vi "Calculate Ascan Parameter.vi"(8 "error in (no error)":errorcluster caption="错误输入（无错误）", 10 "data":T1(array[cluster]), 11 "connection reference":T2) -> (0 "error out":errorcluster caption="错误输出")   [LabVIEW 2015, in "Digital Signal Processing.lvlib"]
doc: "该模板用于创建子VI。"
uses:
  Digital Signal Processing.lvlib
  <vilib>/addons/database/Connection.llb/Conn ObjectReference.ctl
  Utility VIs/Utility VIs.lvlib
  <vilib>/Analysis/NI_AALBase.lvlib
  Database Processing/Database Processing.lvlib
  <vilib>/addons/database/NI_Database_API.lvlib
  Digital Image Processing/Digital Image Processing.lvlib
panel:
  # "Busy"
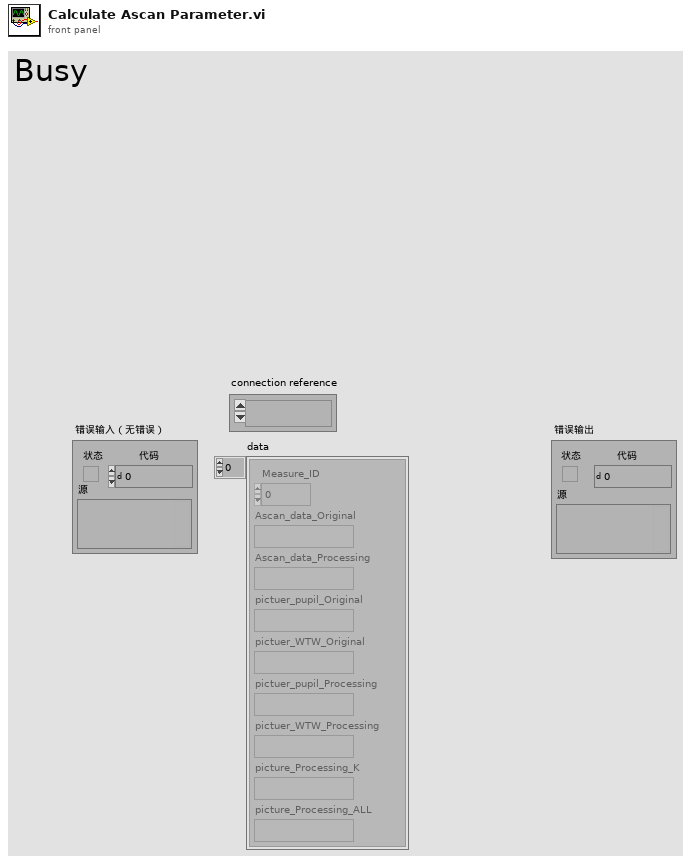
[diagram p1: front panel]
types:
  T1 = cluster{"Measure_ID":i64, "Ascan_data_Original":string, "Ascan_data_Processing":string, "pictuer_pupil_Original":string, "pictuer_WTW_Original":string, "pictuer_pupil_Processing":string, "pictuer_WTW_Processing":string, "picture_Processing_K":string, "picture_Processing_ALL":string}[]
  T2 = typedef "NI_Database_API.lvlib/Conn ObjectReference.ctl" = refnum<k1>
  T3 = cluster{"Measure_ID":i64, "Ascan_data_Original":string, "Ascan_data_Processing":string, "pictuer_pupil_Original":string, "pictuer_WTW_Original":string, "pictuer_pupil_Processing":string, "pictuer_WTW_Processing":string, "picture_Processing_K":string, "picture_Processing_ALL":string}
  T4 = typedef "Digital Signal Processing.lvlib/DSP Configuration.ctl" = cluster{"Sampling Frequency":dbl, "filter type":T5, "RF Filter Low Frequency":dbl, "RF Filter High Frequency":dbl, "RF Filter Taps":i32, "window":T6, "RF window parameter":dbl, "filter type 2":T5, "Demodulated Filter Low Frequency":dbl, "Demodulated Filter HighFrequency":dbl, "Demodulated Filter Order":i32, "SPAN":i32, "Logarithmic Base":dbl, "Noise path":string, "Work position parameter":i32[]}
  T5 = typedef "NI_AALBase.lvlib/Filter Passband Type.ctl" = enum32{"Lowpass", "Highpass", "Bandpass", "Bandstop"}
  T6 = typedef "NI_AALPro.lvlib/windowTd.ctl" = u32
  T7 = cluster{"filter structure":enum32{"IIR 2nd Order", "IIR 4th Order"}, "Reverse Coefficients":dbl[], "Forward Coefficients":dbl[]}
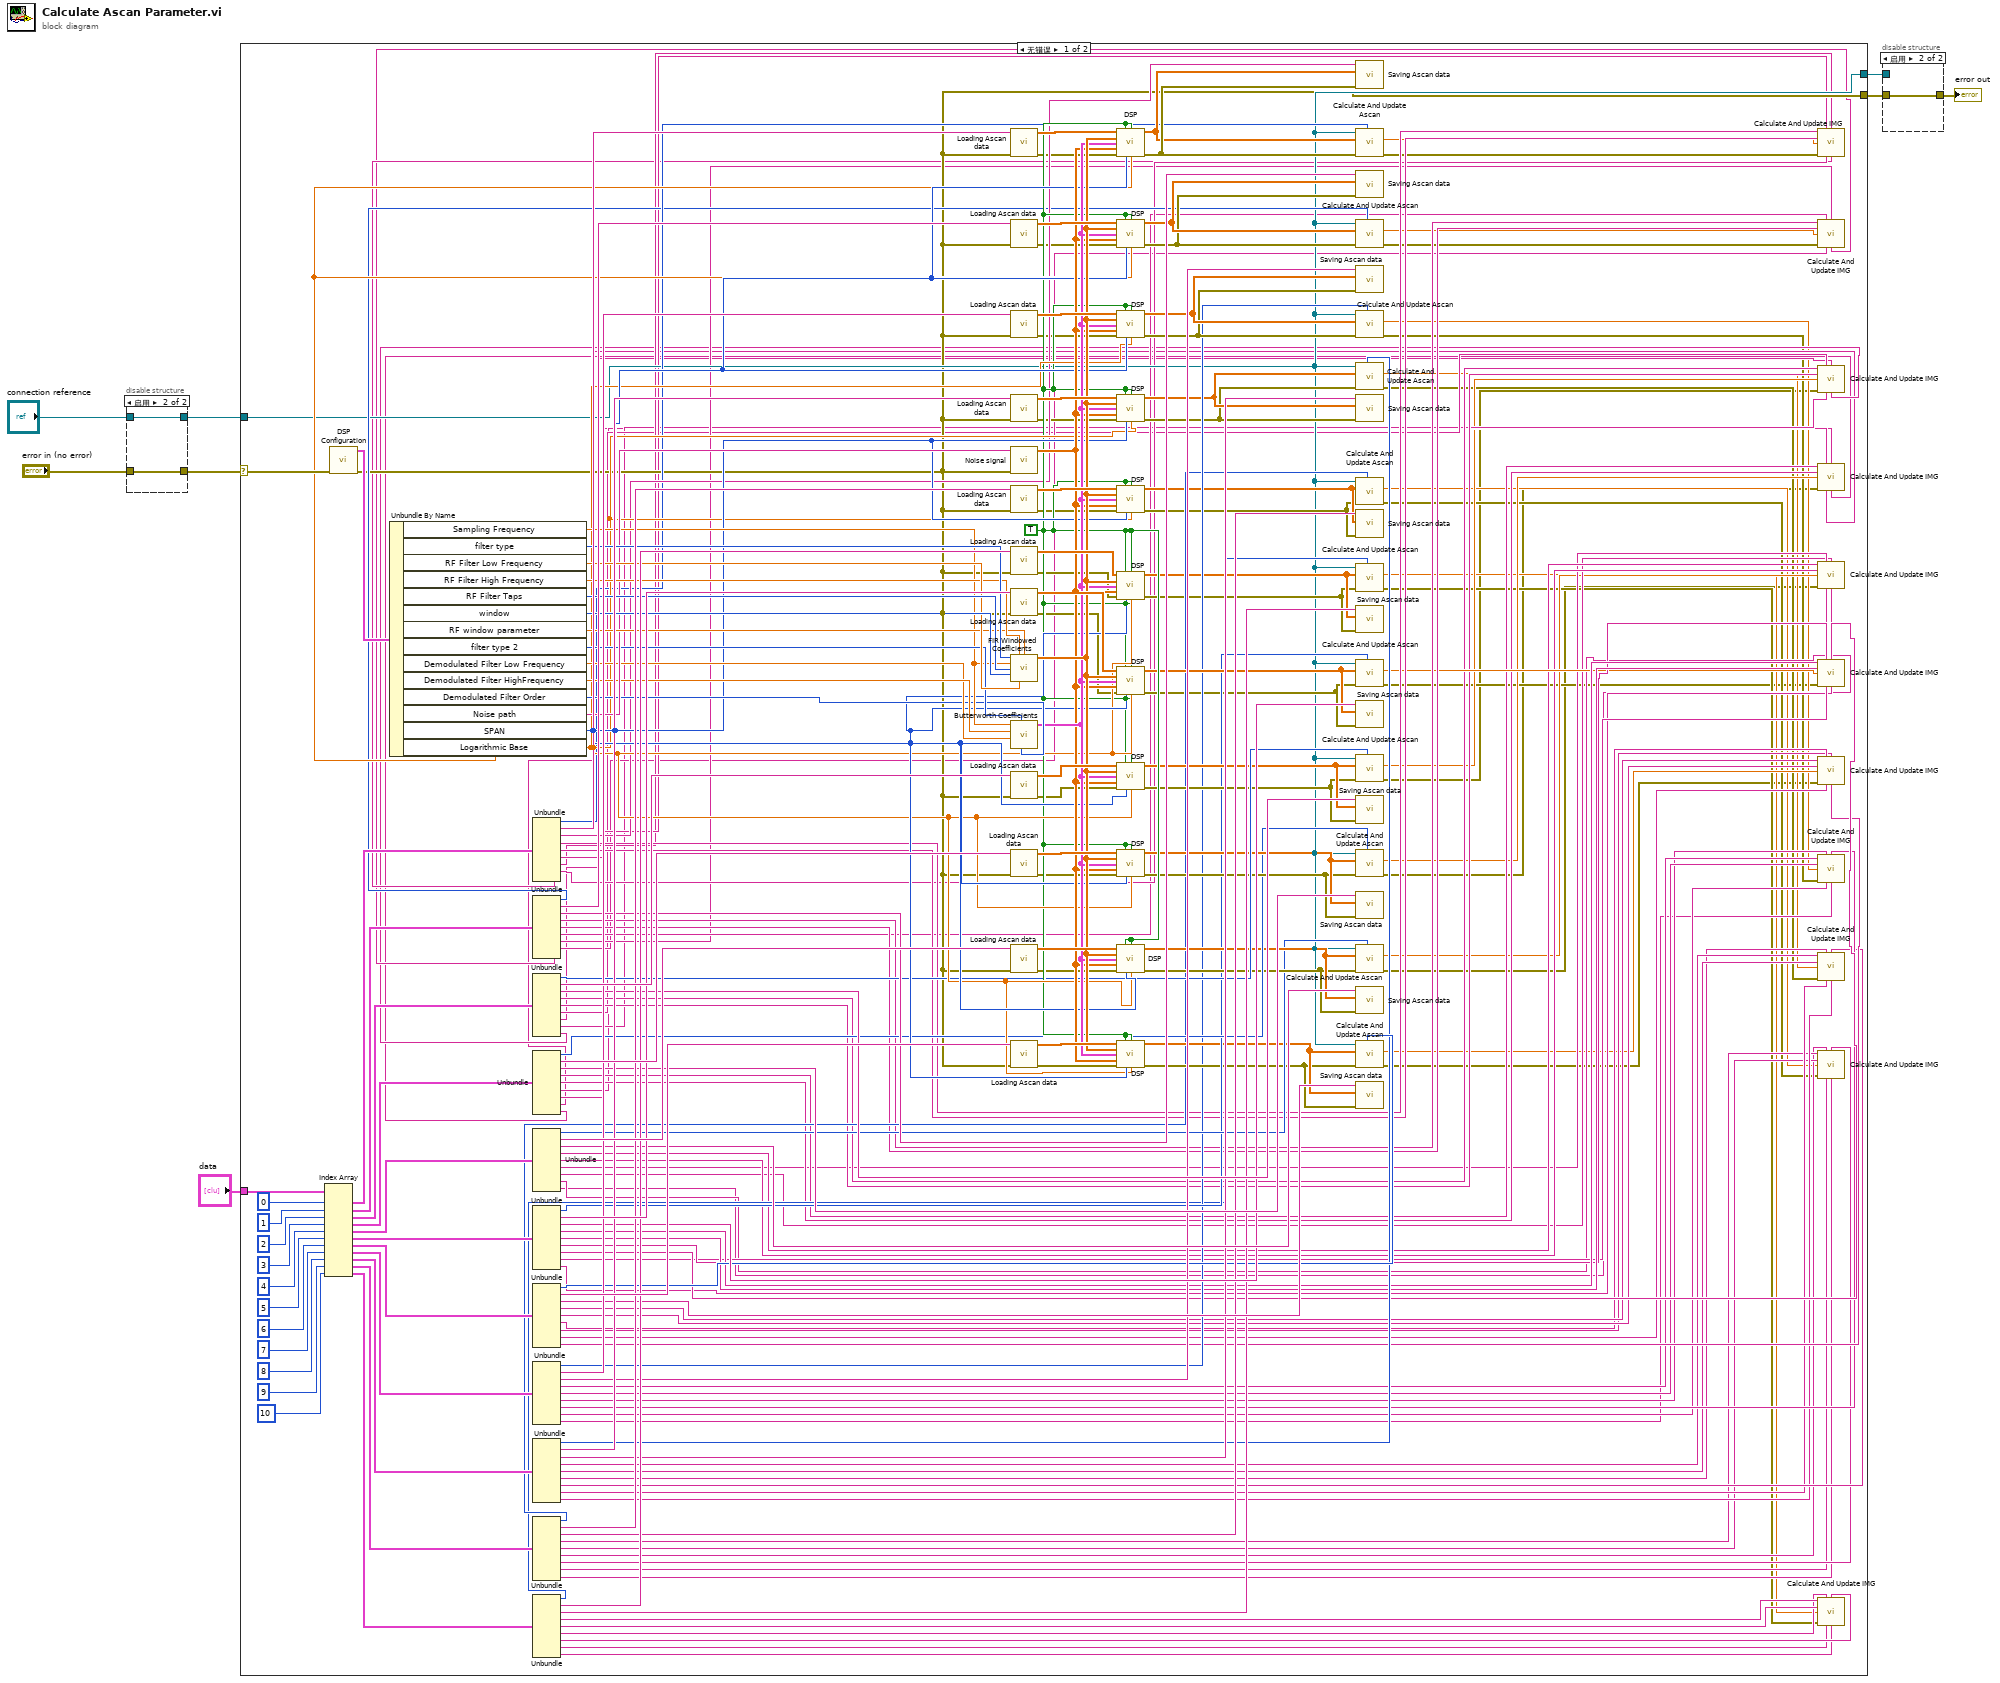
[diagram p0: block diagram]
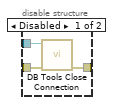
[diagram p2: hidden frame]
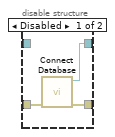
[diagram p3: hidden frame]
diagram:
  n1 = disable-structure shown="启用" {
    disable-tunnel: [w11 w13] -> w8
    disable-tunnel: "error in (no error)" -> [w10 w12]
    disable-tunnel: [w9 w12] -> w6
    disable-tunnel: "connection reference" -> [_ w13]
    frame Disabled {
      n2 = call "Connect Database.vi"("error in (no error)"=w10) -> ("error out"=w9:errorcluster, "connection reference"=w11:T2)  [unwired: 9 in]
    }
    frame Enabled {
    }
  }
  n3 = case shown="无错误" w6 {
    selector: w6 -> [w166 w225]
    tunnel: [w102 w225] -> w4
    tunnel: "data" -> [w223 _]
    tunnel: w8 -> [w103 w224]
    tunnel: [w103 w224] -> w2
    frame No Error {
      w159 = TRUE
      n4 = Index Array(array=w223, index #1=0 ("索引"), index #2=1 ("索引"), index #3=2 ("索引"), index #4=3 ("索引"), index #5=4 ("索引"), index #6=5 ("索引"), index #7=6 ("索引"), index #8=7 ("索引"), index #9=8 ("索引"), index #10=9 ("索引"), index #11=10 ("索引")) -> (element #1=w211:T3, element #2=w201:T3, element #3=w200:T3, element #4=w199:T3, element #5=w198:T3, element #6=w197:T3, element #7=w196:T3, element #8=w195:T3, element #9=w194:T3, element #10=w191:T3, element #11=w190:T3)
      n5 = call "DSP Configuration.vi"("error in (no error)"=w166) -> ("error out"=w102:errorcluster, "DSP Parameter Output"=w165:T4)  [unwired: 9 in]
      n6 = Unbundle By Name(w165) -> ("Sampling Frequency"=w170:dbl, "filter type"=w178:T5, "RF Filter Low Frequency"=w175:dbl, "RF Filter High Frequency"=w174:dbl, "RF Filter Taps"=w177:i32, "window"=w176:T6, "RF window parameter"=w173:dbl, "filter type 2"=w171:T5, "Demodulated Filter Low Frequency"=w168:dbl, "Demodulated Filter HighFrequency"=w169:dbl, "Demodulated Filter Order"=w167:i32, "Noise path"=w172:string, "SPAN"=w161:i32, "Logarithmic Base"=w160:dbl)
      n7 = Unbundle(w211) -> ("Measure_ID"=w134:i64, "Ascan_data_Original"=w210:string, "Ascan_data_Processing"=w158:string, "pictuer_pupil_Original"=w101:string, "pictuer_WTW_Original"=w100:string, "pictuer_pupil_Processing"=w99:string, "pictuer_WTW_Processing"=w98:string, "picture_Processing_K"=w97:string, "picture_Processing_ALL"=w96:string)
      n8 = Unbundle(w201) -> ("Measure_ID"=w131:i64, "Ascan_data_Original"=w209:string, "Ascan_data_Processing"=w157:string, "pictuer_pupil_Original"=w93:string, "pictuer_WTW_Original"=w92:string, "pictuer_pupil_Processing"=w91:string, "pictuer_WTW_Processing"=w90:string, "picture_Processing_K"=w89:string, "picture_Processing_ALL"=w88:string)
      n9 = Unbundle(w200) -> ("Measure_ID"=w130:i64, "Ascan_data_Original"=w208:string, "Ascan_data_Processing"=w156:string, "pictuer_pupil_Original"=w78:string, "pictuer_WTW_Original"=w77:string, "pictuer_pupil_Processing"=w76:string, "pictuer_WTW_Processing"=w75:string, "picture_Processing_K"=w74:string, "picture_Processing_ALL"=w73:string)
      n10 = Unbundle(w199) -> ("Measure_ID"=w125:i64, "Ascan_data_Original"=w207:string, "Ascan_data_Processing"=w155:string, "pictuer_pupil_Original"=w72:string, "pictuer_WTW_Original"=w71:string, "pictuer_pupil_Processing"=w70:string, "pictuer_WTW_Processing"=w69:string, "picture_Processing_K"=w68:string, "picture_Processing_ALL"=w67:string)
      n11 = Unbundle(w198) -> ("Measure_ID"=w122:i64, "Ascan_data_Original"=w206:string, "Ascan_data_Processing"=w154:string, "pictuer_pupil_Original"=w65:string, "pictuer_WTW_Original"=w64:string, "pictuer_pupil_Processing"=w63:string, "pictuer_WTW_Processing"=w62:string, "picture_Processing_K"=w61:string, "picture_Processing_ALL"=w60:string)
      n12 = Unbundle(w197) -> ("Measure_ID"=w120:i64, "Ascan_data_Original"=w205:string, "Ascan_data_Processing"=w153:string, "pictuer_pupil_Original"=w85:string, "pictuer_WTW_Original"=w84:string, "pictuer_pupil_Processing"=w83:string, "pictuer_WTW_Processing"=w82:string, "picture_Processing_K"=w81:string, "picture_Processing_ALL"=w80:string)
      n13 = Unbundle(w196) -> ("Measure_ID"=w119:i64, "Ascan_data_Original"=w204:string, "Ascan_data_Processing"=w152:string, "pictuer_pupil_Original"=w59:string, "pictuer_WTW_Original"=w58:string, "pictuer_pupil_Processing"=w57:string, "pictuer_WTW_Processing"=w56:string, "picture_Processing_K"=w55:string, "picture_Processing_ALL"=w54:string)
      n14 = Unbundle(w195) -> ("Measure_ID"=w114:i64, "Ascan_data_Original"=w203:string, "Ascan_data_Processing"=w151:string, "pictuer_pupil_Original"=w53:string, "pictuer_WTW_Original"=w52:string, "pictuer_pupil_Processing"=w51:string, "pictuer_WTW_Processing"=w50:string, "picture_Processing_K"=w49:string, "picture_Processing_ALL"=w48:string)
      n15 = Unbundle(w194) -> ("Measure_ID"=w113:i64, "Ascan_data_Original"=w202:string, "Ascan_data_Processing"=w150:string, "pictuer_pupil_Original"=w47:string, "pictuer_WTW_Original"=w46:string, "pictuer_pupil_Processing"=w45:string, "pictuer_WTW_Processing"=w44:string, "picture_Processing_K"=w43:string, "picture_Processing_ALL"=w42:string)
      n16 = Unbundle(w191) -> ("Measure_ID"=w110:i64, "Ascan_data_Original"=w193:string, "Ascan_data_Processing"=w149:string, "pictuer_pupil_Original"=w41:string, "pictuer_WTW_Original"=w40:string, "pictuer_pupil_Processing"=w39:string, "pictuer_WTW_Processing"=w38:string, "picture_Processing_K"=w37:string, "picture_Processing_ALL"=w36:string)
      n17 = Unbundle(w190) -> ("Measure_ID"=w105:i64, "Ascan_data_Original"=w192:string, "Ascan_data_Processing"=w148:string, "pictuer_pupil_Original"=w35:string, "pictuer_WTW_Original"=w34:string, "pictuer_pupil_Processing"=w33:string, "pictuer_WTW_Processing"=w32:string, "picture_Processing_K"=w31:string, "picture_Processing_ALL"=w30:string)
      n18 = call "Loading Ascan data.vi"("error in (no error)"=w102, "名称或相对路径"=w210) -> ("error out"=w147:errorcluster, "first row"=w189:dbl[])  [unwired: 8 in]
      n19 = call "Loading Ascan data.vi"("error in (no error)"=w102, "名称或相对路径"=w209) -> ("error out"=w146:errorcluster, "first row"=w188:dbl[])  [unwired: 8 in]
      n20 = call "Loading Ascan data.vi"("error in (no error)"=w102, "名称或相对路径"=w203) -> ("error out"=w140:errorcluster, "first row"=w182:dbl[])  [unwired: 8 in]
      n21 = call "Loading Ascan data.vi"("error in (no error)"=w102, "名称或相对路径"=w202) -> ("error out"=w139:errorcluster, "first row"=w181:dbl[])  [unwired: 8 in]
      n22 = call "Noise signal.vi"("错误输入"=w102, "Path"=w172) -> ("output signal"=w162:dbl[])  [unwired: 8 in, 1 out]
      n23 = call "Loading Ascan data.vi"("error in (no error)"=w102, "名称或相对路径"=w193) -> ("error out"=w138:errorcluster, "first row"=w180:dbl[])  [unwired: 8 in]
      n24 = call "Loading Ascan data.vi"("error in (no error)"=w102, "名称或相对路径"=w192) -> ("error out"=w137:errorcluster, "first row"=w179:dbl[])  [unwired: 8 in]
      n25 = call "Loading Ascan data.vi"("error in (no error)"=w102, "名称或相对路径"=w205) -> ("error out"=w142:errorcluster, "first row"=w184:dbl[])  [unwired: 8 in]
      n26 = call <vilib>:"FIR Windowed Coefficients.vi"("filter type"=w178, "high cutoff freq: fh"=w174, "window parameter"=w173, "sampling freq: fs"=w170, "taps"=w177, "window"=w176, "low cutoff freq: fl"=w175) -> ("FIR Windowed Coefficients"=w164:dbl[])  [unwired: 1 in, 7 out]
      n27 = call <vilib>:"Butterworth Coefficients.vi"("order"=w167, "filter type"=w171, "low cutoff freq: fl"=w168, "high cutoff freq: fh"=w169, "sampling freq: fs"=w170) -> ("IIR Filter Cluster"=w163:T7)  [unwired: 5 in, 1 out]
      n28 = call "Loading Ascan data.vi"("error in (no error)"=w102, "名称或相对路径"=w208) -> ("error out"=w145:errorcluster, "first row"=w187:dbl[])  [unwired: 8 in]
      n29 = call "Loading Ascan data.vi"("error in (no error)"=w102, "名称或相对路径"=w207) -> ("error out"=w144:errorcluster, "first row"=w186:dbl[])  [unwired: 8 in]
      n30 = call "Loading Ascan data.vi"("error in (no error)"=w102, "名称或相对路径"=w206) -> ("error out"=w143:errorcluster, "first row"=w185:dbl[])  [unwired: 8 in]
      n31 = call "Loading Ascan data.vi"("error in (no error)"=w102, "名称或相对路径"=w204) -> ("error out"=w141:errorcluster, "first row"=w183:dbl[])  [unwired: 8 in]
      n32 = call "DSP.vi"("Input Signal"=w189, "Smooth(F : Don't)"=w159, "Minus Noise(F : Don't)"=w159, "RF Window"=w164, "IIR Filter Cluster"=w163, "Noise Signal"=w162, "error in (no error)"=w147, "SPAN"=w161, "Logarithmic Base"=w160) -> ("DSP signal"=w135:dbl[], "error out"=w136:errorcluster)  [unwired: 5 in]
      n33 = call "DSP.vi"("Input Signal"=w188, "Smooth(F : Don't)"=w159, "Minus Noise(F : Don't)"=w159, "RF Window"=w164, "IIR Filter Cluster"=w163, "Noise Signal"=w162, "error in (no error)"=w146, "SPAN"=w161, "Logarithmic Base"=w160) -> ("DSP signal"=w133:dbl[], "error out"=w132:errorcluster)  [unwired: 5 in]
      n34 = call "DSP.vi"("Input Signal"=w182, "Smooth(F : Don't)"=w159, "Minus Noise(F : Don't)"=w159, "RF Window"=w164, "IIR Filter Cluster"=w163, "Noise Signal"=w162, "error in (no error)"=w140, "SPAN"=w161, "Logarithmic Base"=w160) -> ("DSP signal"=w116:dbl[], "error out"=w115:errorcluster)  [unwired: 5 in]
      n35 = call "DSP.vi"("Input Signal"=w181, "Smooth(F : Don't)"=w159, "Minus Noise(F : Don't)"=w159, "RF Window"=w164, "IIR Filter Cluster"=w163, "Noise Signal"=w162, "error in (no error)"=w139, "SPAN"=w161, "Logarithmic Base"=w160) -> ("DSP signal"=w112:dbl[], "error out"=w111:errorcluster)  [unwired: 5 in]
      n36 = call "DSP.vi"("Input Signal"=w180, "Smooth(F : Don't)"=w159, "Minus Noise(F : Don't)"=w159, "RF Window"=w164, "IIR Filter Cluster"=w163, "Noise Signal"=w162, "error in (no error)"=w138, "SPAN"=w161, "Logarithmic Base"=w160) -> ("DSP signal"=w109:dbl[], "error out"=w108:errorcluster)  [unwired: 5 in]
      n37 = call "DSP.vi"("Input Signal"=w179, "Smooth(F : Don't)"=w159, "Minus Noise(F : Don't)"=w159, "RF Window"=w164, "IIR Filter Cluster"=w163, "Noise Signal"=w162, "error in (no error)"=w137, "SPAN"=w161, "Logarithmic Base"=w160) -> ("DSP signal"=w107:dbl[], "error out"=w106:errorcluster)  [unwired: 5 in]
      n38 = call "DSP.vi"("Input Signal"=w184, "Smooth(F : Don't)"=w159, "Minus Noise(F : Don't)"=w159, "RF Window"=w164, "IIR Filter Cluster"=w163, "Noise Signal"=w162, "error in (no error)"=w142, "SPAN"=w161, "Logarithmic Base"=w160) -> ("DSP signal"=w121:dbl[], "error out"=w104:errorcluster)  [unwired: 5 in]
      n39 = call "DSP.vi"("Input Signal"=w187, "Smooth(F : Don't)"=w159, "Minus Noise(F : Don't)"=w159, "RF Window"=w164, "IIR Filter Cluster"=w163, "Noise Signal"=w162, "error in (no error)"=w145, "SPAN"=w161, "Logarithmic Base"=w160) -> ("DSP signal"=w129:dbl[], "error out"=w128:errorcluster)  [unwired: 5 in]
      n40 = call "DSP.vi"("Input Signal"=w186, "Smooth(F : Don't)"=w159, "Minus Noise(F : Don't)"=w159, "RF Window"=w164, "IIR Filter Cluster"=w163, "Noise Signal"=w162, "error in (no error)"=w144, "SPAN"=w161, "Logarithmic Base"=w160) -> ("DSP signal"=w127:dbl[], "error out"=w126:errorcluster)  [unwired: 5 in]
      n41 = call "DSP.vi"("Input Signal"=w185, "Smooth(F : Don't)"=w159, "Minus Noise(F : Don't)"=w159, "RF Window"=w164, "IIR Filter Cluster"=w163, "Noise Signal"=w162, "error in (no error)"=w143, "SPAN"=w161, "Logarithmic Base"=w160) -> ("DSP signal"=w124:dbl[], "error out"=w123:errorcluster)  [unwired: 5 in]
      n42 = call "DSP.vi"("Input Signal"=w183, "Smooth(F : Don't)"=w159, "Minus Noise(F : Don't)"=w159, "RF Window"=w164, "IIR Filter Cluster"=w163, "Noise Signal"=w162, "error in (no error)"=w141, "SPAN"=w161, "Logarithmic Base"=w160) -> ("DSP signal"=w118:dbl[], "error out"=w117:errorcluster)  [unwired: 5 in]
      n43 = call "Saving Ascan data.vi"("error in (no error)"=w136, "Ascan Data"=w135, "名称或相对路径"=w158) -> ()  [unwired: 8 in, 1 out]
      n44 = call "Calculate And Update Ascan.vi"("Measure_ID"=w134, "error in (no error)"=w136, "S"=w135, "connection reference"=w103) -> ("error out"=w94:errorcluster, "开始位置"=w95:dbl)  [unwired: 6 in]
      n45 = call "Saving Ascan data.vi"("error in (no error)"=w132, "Ascan Data"=w133, "名称或相对路径"=w157) -> ()  [unwired: 8 in, 1 out]
      n46 = call "Calculate And Update Ascan.vi"("Measure_ID"=w131, "error in (no error)"=w132, "S"=w133, "connection reference"=w103) -> ("error out"=w86:errorcluster, "开始位置"=w87:dbl)  [unwired: 6 in]
      n47 = call "Saving Ascan data.vi"("error in (no error)"=w115, "Ascan Data"=w116, "名称或相对路径"=w151) -> ()  [unwired: 8 in, 1 out]
      n48 = call "Calculate And Update Ascan.vi"("Measure_ID"=w114, "error in (no error)"=w115, "S"=w116, "connection reference"=w103) -> ("error out"=w21:errorcluster, "开始位置"=w23:dbl)  [unwired: 6 in]
      n49 = call "Calculate And Update Ascan.vi"("Measure_ID"=w113, "error in (no error)"=w111, "S"=w112, "connection reference"=w103) -> ("error out"=w22:errorcluster, "开始位置"=w24:dbl)  [unwired: 6 in]
      n50 = call "Saving Ascan data.vi"("error in (no error)"=w111, "Ascan Data"=w112, "名称或相对路径"=w150) -> ()  [unwired: 8 in, 1 out]
      n51 = call "Calculate And Update Ascan.vi"("Measure_ID"=w110, "error in (no error)"=w108, "S"=w109, "connection reference"=w103) -> ("error out"=w20:errorcluster, "开始位置"=w25:dbl)  [unwired: 6 in]
      n52 = call "Saving Ascan data.vi"("error in (no error)"=w108, "Ascan Data"=w109, "名称或相对路径"=w149) -> ()  [unwired: 8 in, 1 out]
      n53 = call "Calculate And Update Ascan.vi"("Measure_ID"=w105, "error in (no error)"=w106, "S"=w107, "connection reference"=w103) -> ("error out"=w19:errorcluster, "开始位置"=w26:dbl)  [unwired: 6 in]
      n54 = call "Saving Ascan data.vi"("error in (no error)"=w106, "Ascan Data"=w107, "名称或相对路径"=w148) -> ()  [unwired: 8 in, 1 out]
      n55 = call "Calculate And Update Ascan.vi"("Measure_ID"=w120, "error in (no error)"=w104, "S"=w121, "connection reference"=w103) -> ("error out"=w18:errorcluster, "开始位置"=w79:dbl)  [unwired: 6 in]
      n56 = call "Saving Ascan data.vi"("error in (no error)"=w104, "Ascan Data"=w121, "名称或相对路径"=w153) -> ()  [unwired: 8 in, 1 out]
      n57 = call "Calculate And Update Ascan.vi"("Measure_ID"=w130, "error in (no error)"=w128, "S"=w129, "connection reference"=w103) -> ("error out"=w17:errorcluster, "开始位置"=w66:dbl)  [unwired: 6 in]
      n58 = call "Saving Ascan data.vi"("error in (no error)"=w128, "Ascan Data"=w129, "名称或相对路径"=w156) -> ()  [unwired: 8 in, 1 out]
      n59 = call "Calculate And Update Ascan.vi"("Measure_ID"=w125, "error in (no error)"=w126, "S"=w127, "connection reference"=w103) -> ("error out"=w16:errorcluster, "开始位置"=w27:dbl)  [unwired: 6 in]
      n60 = call "Saving Ascan data.vi"("error in (no error)"=w126, "Ascan Data"=w127, "名称或相对路径"=w155) -> ()  [unwired: 8 in, 1 out]
      n61 = call "Calculate And Update Ascan.vi"("Measure_ID"=w122, "error in (no error)"=w123, "S"=w124, "connection reference"=w103) -> ("error out"=w15:errorcluster, "开始位置"=w28:dbl)  [unwired: 6 in]
      n62 = call "Saving Ascan data.vi"("error in (no error)"=w123, "Ascan Data"=w124, "名称或相对路径"=w154) -> ()  [unwired: 8 in, 1 out]
      n63 = call "Calculate And Update Ascan.vi"("Measure_ID"=w119, "error in (no error)"=w117, "S"=w118, "connection reference"=w103) -> ("error out"=w14:errorcluster, "开始位置"=w29:dbl)  [unwired: 6 in]
      n64 = call "Saving Ascan data.vi"("error in (no error)"=w117, "Ascan Data"=w118, "名称或相对路径"=w152) -> ()  [unwired: 8 in, 1 out]
      n65 = call "Calculate And Update IMG.vi"("pictuer_pupil_Original"=w101, "pictuer_pupil_Processing"=w99, "pictuer_WTW_Processing"=w98, "pictuer_WTW_Original"=w100, "D"=w95, "error in (no error)"=w94, "picture_Processing_K"=w97, "picture_Processing_ALL"=w96) -> ()  [unwired: 3 in, 5 out]
      n66 = call "Calculate And Update IMG.vi"("pictuer_pupil_Original"=w93, "pictuer_pupil_Processing"=w91, "pictuer_WTW_Processing"=w90, "pictuer_WTW_Original"=w92, "D"=w87, "error in (no error)"=w86, "picture_Processing_K"=w89, "picture_Processing_ALL"=w88) -> ()  [unwired: 3 in, 5 out]
      n67 = call "Calculate And Update IMG.vi"("pictuer_pupil_Original"=w78, "pictuer_pupil_Processing"=w76, "pictuer_WTW_Processing"=w75, "pictuer_WTW_Original"=w77, "D"=w66, "error in (no error)"=w17, "picture_Processing_K"=w74, "picture_Processing_ALL"=w73) -> ()  [unwired: 3 in, 5 out]
      n68 = call "Calculate And Update IMG.vi"("pictuer_pupil_Original"=w72, "pictuer_pupil_Processing"=w70, "pictuer_WTW_Processing"=w69, "pictuer_WTW_Original"=w71, "D"=w27, "error in (no error)"=w16, "picture_Processing_K"=w68, "picture_Processing_ALL"=w67) -> ()  [unwired: 3 in, 5 out]
      n69 = call "Calculate And Update IMG.vi"("pictuer_pupil_Original"=w65, "pictuer_pupil_Processing"=w63, "pictuer_WTW_Processing"=w62, "pictuer_WTW_Original"=w64, "D"=w28, "error in (no error)"=w15, "picture_Processing_K"=w61, "picture_Processing_ALL"=w60) -> ()  [unwired: 3 in, 5 out]
      n70 = call "Calculate And Update IMG.vi"("pictuer_pupil_Original"=w85, "pictuer_pupil_Processing"=w83, "pictuer_WTW_Processing"=w82, "pictuer_WTW_Original"=w84, "D"=w79, "error in (no error)"=w18, "picture_Processing_K"=w81, "picture_Processing_ALL"=w80) -> ()  [unwired: 3 in, 5 out]
      n71 = call "Calculate And Update IMG.vi"("pictuer_pupil_Original"=w59, "pictuer_pupil_Processing"=w57, "pictuer_WTW_Processing"=w56, "pictuer_WTW_Original"=w58, "D"=w29, "error in (no error)"=w14, "picture_Processing_K"=w55, "picture_Processing_ALL"=w54) -> ()  [unwired: 3 in, 5 out]
      n72 = call "Calculate And Update IMG.vi"("pictuer_pupil_Original"=w53, "pictuer_pupil_Processing"=w51, "pictuer_WTW_Processing"=w50, "pictuer_WTW_Original"=w52, "D"=w23, "error in (no error)"=w21, "picture_Processing_K"=w49, "picture_Processing_ALL"=w48) -> ()  [unwired: 3 in, 5 out]
      n73 = call "Calculate And Update IMG.vi"("pictuer_pupil_Original"=w47, "pictuer_pupil_Processing"=w45, "pictuer_WTW_Processing"=w44, "pictuer_WTW_Original"=w46, "D"=w24, "error in (no error)"=w22, "picture_Processing_K"=w43, "picture_Processing_ALL"=w42) -> ()  [unwired: 3 in, 5 out]
      n74 = call "Calculate And Update IMG.vi"("pictuer_pupil_Original"=w41, "pictuer_pupil_Processing"=w39, "pictuer_WTW_Processing"=w38, "pictuer_WTW_Original"=w40, "D"=w25, "error in (no error)"=w20, "picture_Processing_K"=w37, "picture_Processing_ALL"=w36) -> ()  [unwired: 3 in, 5 out]
      n75 = call "Calculate And Update IMG.vi"("pictuer_pupil_Original"=w35, "pictuer_pupil_Processing"=w33, "pictuer_WTW_Processing"=w32, "pictuer_WTW_Original"=w34, "D"=w26, "error in (no error)"=w19, "picture_Processing_K"=w31, "picture_Processing_ALL"=w30) -> ()  [unwired: 3 in, 5 out]
    }
    frame Error {
    }
  }
  n76 = disable-structure shown="启用" {
    disable-tunnel: w4 -> [w228 w229]
    disable-tunnel: [w227 w229] -> w3
    disable-tunnel: w2 -> [w226 _]
    frame Disabled {
      n77 = call <vilib>:"DB Tools Close Connection.vi"("error in (no error)"=w228, "connection reference"=w226) -> ("error out"=w227:errorcluster)  [unwired: 5 in]
    }
    frame Enabled {
    }
  }
  "error out" <- w3
